vi "imu2Angle.vi"(11 "Sensor Input":dbl) -> (3 "Angle (radians)":dbl)   [LabVIEW 2019]
panel:
  in  "Offset":dbl
  in  "Gain":dbl=0.00614
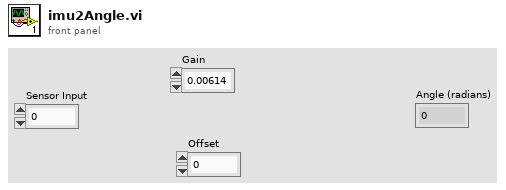
[diagram p1: front panel]
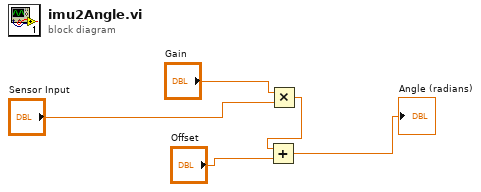
[diagram p0: block diagram]
diagram:
  n1 = Multiply(x="Gain", y="Sensor Input") -> (x*y=w3:dbl)
  n2 = Add(x=w3, y="Offset") -> (x+y=→"Angle (radians)":dbl)
